vi "Add Step Type Specific Results.vi"(6 "Configuration in":refnum<class "Configuration.lvclass">, 8 "error in (no error)":errorcluster, 9 "TestStand Result":T1, 10 "Array in":string[](array[string]), 11 "Result Handler":refnum<class "TestStand Result Handler.lvclass">) -> (0 "error out":errorcluster, 1 "Ignore?":bool, 2 "Array out":string[](array[string]), 3 "Result Handler Out":refnum<class "TestStand Result Handler.lvclass">)   [LabVIEW 2020, in "Astemes_CSVReportPlugin.lvlib" / "TestStand Result Handler.lvclass"]
uses:
  TestStand Result Handler.lvclass
  TestStand Result.ctl
  Configuration/Configuration.lvclass
  Columns.ctl
  TestStand Result Handler.lvclass/TestStand Result Handler.ctl
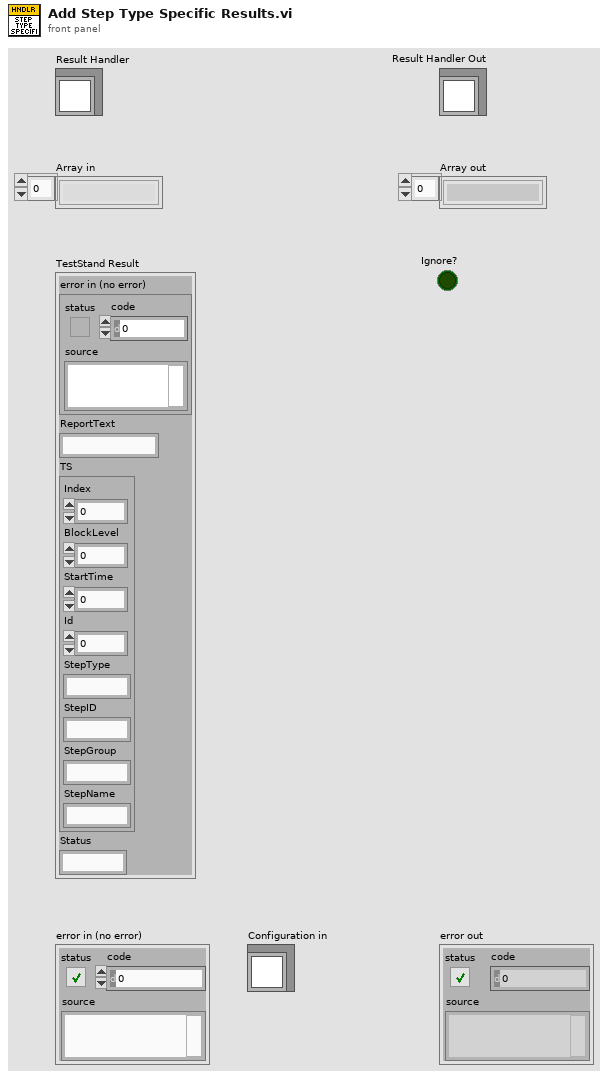
[diagram p1: front panel]
types:
  T1 = typedef "Astemes_CSVReportPlugin.lvlib/TestStand Result Handler.lvclass/TestStand Result.ctl" = cluster{"error in (no error)":errorcluster, "ReportText":string, "TS":cluster{"Index":i32, "BlockLevel":i32, "StartTime":dbl, "Id":i32, "StepType":string, "StepID":string, "StepGroup":string, "StepName":string}, "Status":string}
  T2 = typedef "Astemes_CSVReportPlugin.lvlib/TestStand Result Handler.lvclass/Step Types.ctl" = enum16{"Unknown", "String Value Test", "Numeric Limit Test", "Action", "Flow Control"}
  T3 = typedef "Astemes_CSVReportPlugin.lvlib/TestStand Result Handler.lvclass/Columns.ctl" = enum16{"StepName", "Result", "LowerLimit", "ComparisonTypeLow", "Measurement", "ComparisonTypeHigh", "UpperLimit", "ReportText", "StepType"}
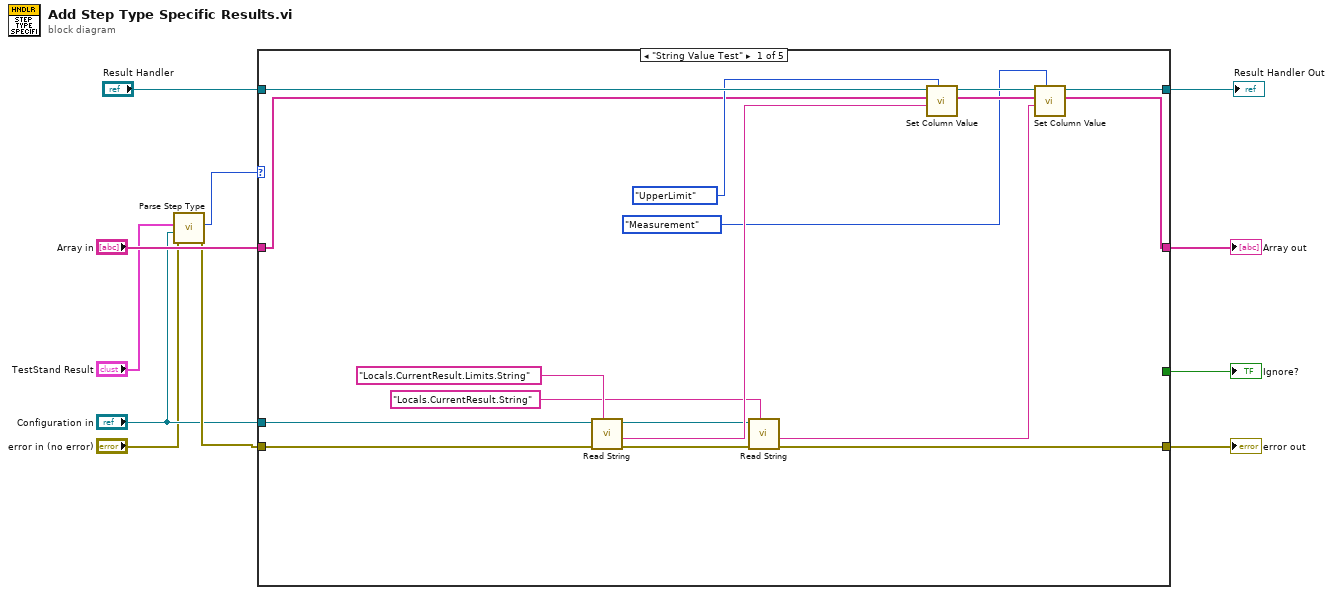
[diagram p0: block diagram]
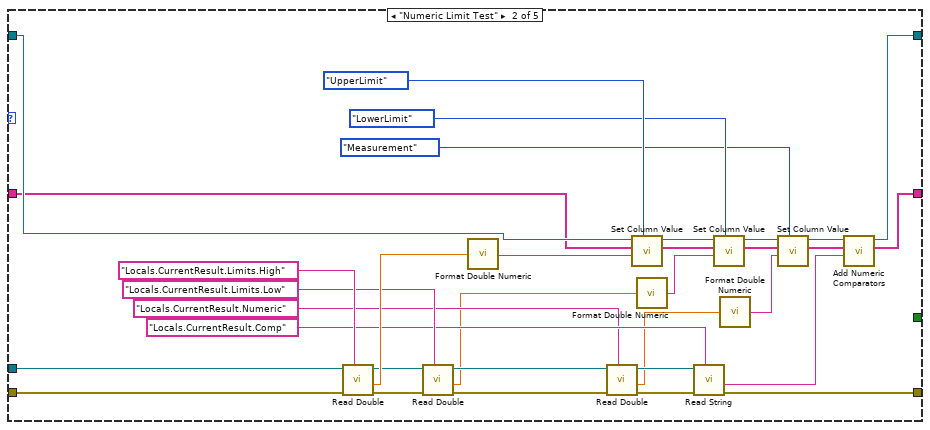
[diagram p2: hidden frame]
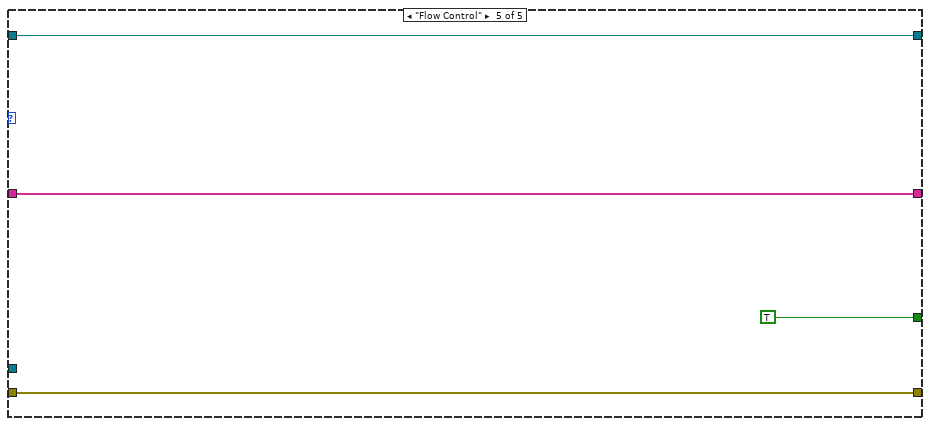
[diagram p5: hidden frame]
diagram:
  n1 = call "Parse Step Type.vi"("error in (no error)"="error in (no error)", "Sequence Context"="Configuration in", "TestStand Result in"="TestStand Result") -> ("error out"=w8:errorcluster, "Step Type"=w6:T2)  [unwired: 7 in]
  n2 = case shown="\"String Value Test\"" w6 {
    tunnel: [w14 w51 w64 w67 w71] -> w5
    tunnel: "Configuration in" -> [w28 w61 _ _ _]
    tunnel: w8 -> [w26 w59 w64 w67 w71]
    tunnel: "Array in" -> [w22 w31 w63 w66 w70]
    tunnel: [w18 w38 w63 w66 w70] -> w11
    tunnel: [_ _ _ _ TRUE] -> w3
    tunnel: "Result Handler" -> [w24 w40 w62 w65 w68]
    tunnel: [w20 w37 w62 w65 w68] -> w1
    frame "String Value Test" {
      n3 = call-dynamic "Read String.vi"("key"="Locals.CurrentResult.Limits.String", "error in (no error)"=w26, "Configuration In"=w28) -> ("error out"=w15:errorcluster, "value"=w25:string, "Configuration Out"=w16:refnum<class "Configuration.lvclass">)  [unwired: 6 in]
      n4 = call-dynamic "Read String.vi"("key"="Locals.CurrentResult.String", "error in (no error)"=w15, "Configuration In"=w16) -> ("error out"=w14:errorcluster, "value"=w12:string)  [unwired: 6 in, 1 out]
      n5 = call "Set Column Value.vi"("Column"=Columns."UpperLimit", "Value"=w25, "Row In"=w22, "Result Handler"=w24) -> ("Row Out"=w19:string[], "Result Handler Out"=w21:refnum<class "TestStand Result Handler.lvclass">)  [unwired: 6 in]
      n6 = call "Set Column Value.vi"("Column"=Columns."Measurement", "Value"=w12, "Row In"=w19, "Result Handler"=w21) -> ("Row Out"=w18:string[], "Result Handler Out"=w20:refnum<class "TestStand Result Handler.lvclass">)  [unwired: 6 in]
    }
    frame "Numeric Limit Test" {
      n7 = call-dynamic "Read Double.vi"("key"="Locals.CurrentResult.Limits.High", "error in (no error)"=w59, "Configuration In"=w61) -> ("error out"=w54:errorcluster, "value"=w58:dbl, "Configuration Out"=w55:refnum<class "Configuration.lvclass">)  [unwired: 6 in]
      n8 = call-dynamic "Read Double.vi"("key"="Locals.CurrentResult.Limits.Low", "error in (no error)"=w54, "Configuration In"=w55) -> ("error out"=w53:errorcluster, "value"=w44:dbl, "Configuration Out"=w47:refnum<class "Configuration.lvclass">)  [unwired: 6 in]
      n9 = call "Format Double Numeric.vi"("value"=w58) -> ("String"=w57:string)
      n10 = call-dynamic "Read Double.vi"("key"="Locals.CurrentResult.Numeric", "error in (no error)"=w53, "Configuration In"=w47) -> ("error out"=w48:errorcluster, "value"=w42:dbl, "Configuration Out"=w46:refnum<class "Configuration.lvclass">)  [unwired: 6 in]
      n11 = call "Set Column Value.vi"("Column"=Columns."UpperLimit", "Value"=w57, "Row In"=w31, "Result Handler"=w40) -> ("Row Out"=w32:string[], "Result Handler Out"=w56:refnum<class "TestStand Result Handler.lvclass">)  [unwired: 6 in]
      n12 = call "Format Double Numeric.vi"("value"=w44) -> ("String"=w43:string)
      n13 = call-dynamic "Read String.vi"("key"="Locals.CurrentResult.Comp", "error in (no error)"=w48, "Configuration In"=w46) -> ("error out"=w51:errorcluster, "value"=w39:string)  [unwired: 6 in, 1 out]
      n14 = call "Set Column Value.vi"("Column"=Columns."LowerLimit", "Value"=w43, "Row In"=w32, "Result Handler"=w56) -> ("Row Out"=w29:string[], "Result Handler Out"=w49:refnum<class "TestStand Result Handler.lvclass">)  [unwired: 6 in]
      n15 = call "Format Double Numeric.vi"("value"=w42) -> ("String"=w41:string)
      n16 = call "Set Column Value.vi"("Column"=Columns."Measurement", "Value"=w41, "Row In"=w29, "Result Handler"=w49) -> ("Row Out"=w30:string[], "Result Handler Out"=w33:refnum<class "TestStand Result Handler.lvclass">)  [unwired: 6 in]
      n17 = call "Add Numeric Comparators.vi"("Comparison"=w39, "Array in"=w30, "Result Handler"=w33) -> ("Array out"=w38:string[], "Result Handler Out"=w37:refnum<class "TestStand Result Handler.lvclass">)  [unwired: 7 in]
    }
    frame "Action" {
    }
    frame "Unknown" {
    }
    frame "Flow Control" {
    }
  }
  "Array out" <- w11
  "error out" <- w5
  "Ignore?" <- w3
  "Result Handler Out" <- w1
